vi "demux1-10(x6).vi"   [LabVIEW 2018]
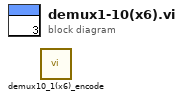
[diagram p0: block diagram]
diagram:
  n1 = call "demux10_1(x6)_encode.vi"() -> ()  [unwired: 10 in, 2 out]
